vi "Generated Descriptors.vi"() -> (3 "Descriptor Strings":string[](array[string]))   [LabVIEW 2019, in "Micron_server.lvlib"]
uses:
  Micron_server.lvlib
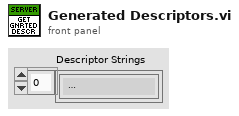
[diagram p1: front panel]
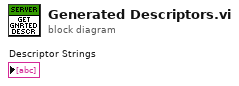
[diagram p0: block diagram]
diagram:
